vi "PicoErrorHandler2.vi"(8 "error in (no error)":errorcluster={"status"=TRUE, "code"=1, "source"="Default Error In"}, 10 "Default handle":i16=16384, 11 "handle In":i16=16384) -> (0 "error out":errorcluster={"status"=TRUE, "code"=1, "source"="Default Error Out"})   [LabVIEW 2020]
doc: "This VI takes an error cluster and if an error has occurred, displays a message box indicating the source of the error and the status code returned by the driver."
uses:
  ps3000a.dll
  ps2000.dll
  ps4000.dll
  ps5000.dll
  ps3000.dll
  ps6000a.dll
  UsbPT104.dll
  ps2000a.dll
  ps5000a.dll
  ps4000a.dll
  ps6000.dll
  plcm3.dll
panel:
  out "CloseUnit Statuses":T1
  out "Pass or Unknown string":string
  out "Error String":string
  out "handle out":i16=16384
  in  "no error":errorcluster
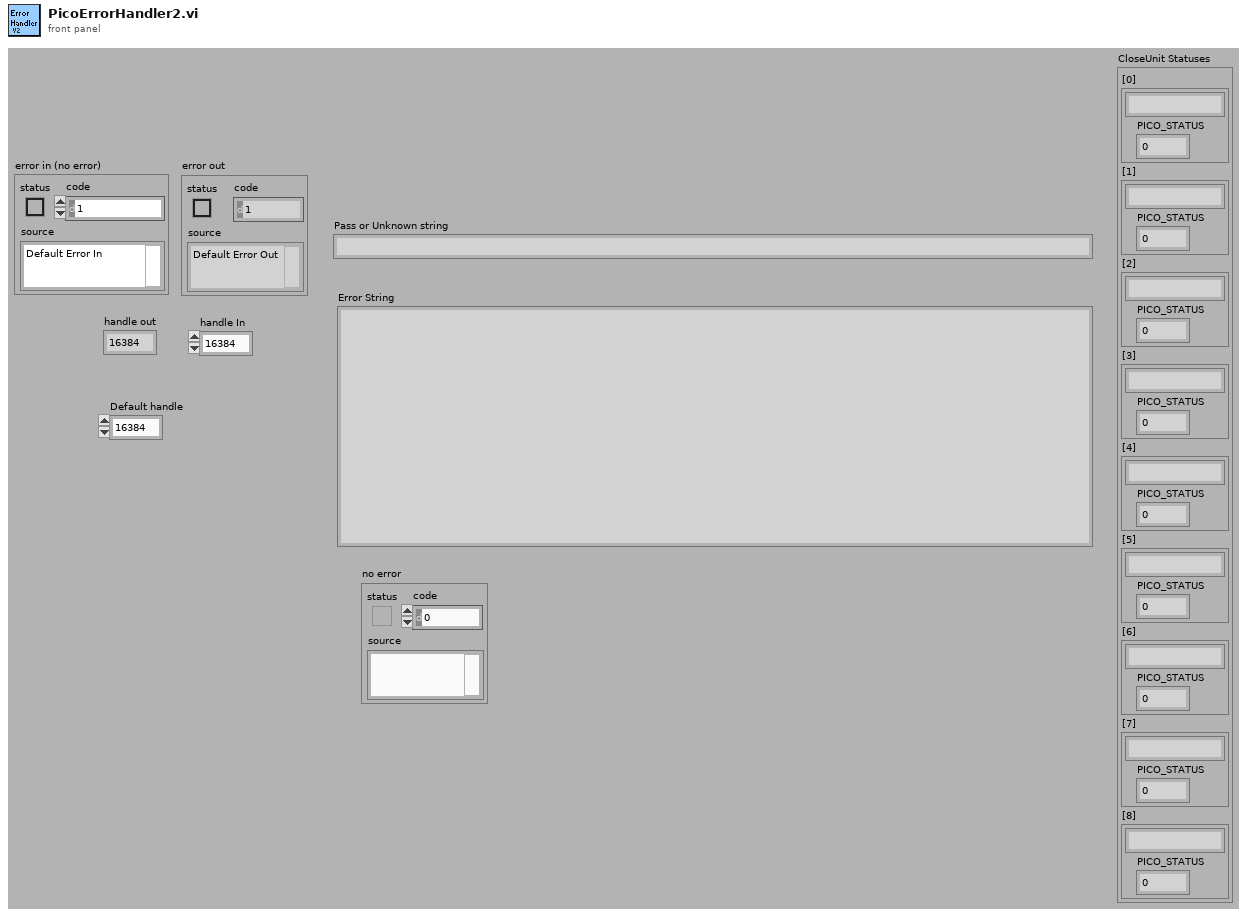
[diagram p1: front panel]
types:
  T1 = cluster{"[0]":cluster{string, "PICO_STATUS":u32}, "[1]":cluster{string, "PICO_STATUS":u32}, "[2]":cluster{string, "PICO_STATUS":u32}, "[3]":cluster{string, "PICO_STATUS":u32}, "[4]":cluster{string, "PICO_STATUS":u32}, "[5]":cluster{string, "PICO_STATUS":u32}, "[6]":cluster{string, "PICO_STATUS":u32}, "[7]":cluster{string, "PICO_STATUS":u32}, "[8]":cluster{string, "PICO_STATUS":u32}}
  T2 = enum16{"Left Button", "Center Button", "Right Button", "Window Close"}
  T3 = cluster{"[0]":cluster{"source":string, "PICO_STATUS":u32}, "[1]":cluster{"source":string, "PICO_STATUS":u32}, "[2]":cluster{"source":string, "PICO_STATUS":u32}, "[3]":cluster{"source":string, "PICO_STATUS":u32}, "[4]":cluster{"source":string, "PICO_STATUS":u32}, "[5]":cluster{"source":string, "PICO_STATUS":u32}, "[6]":cluster{"source":string, "PICO_STATUS":u32}, "[7]":cluster{"source":string, "PICO_STATUS":u32}, "[8]":cluster{"source":string, "PICO_STATUS":u32}}
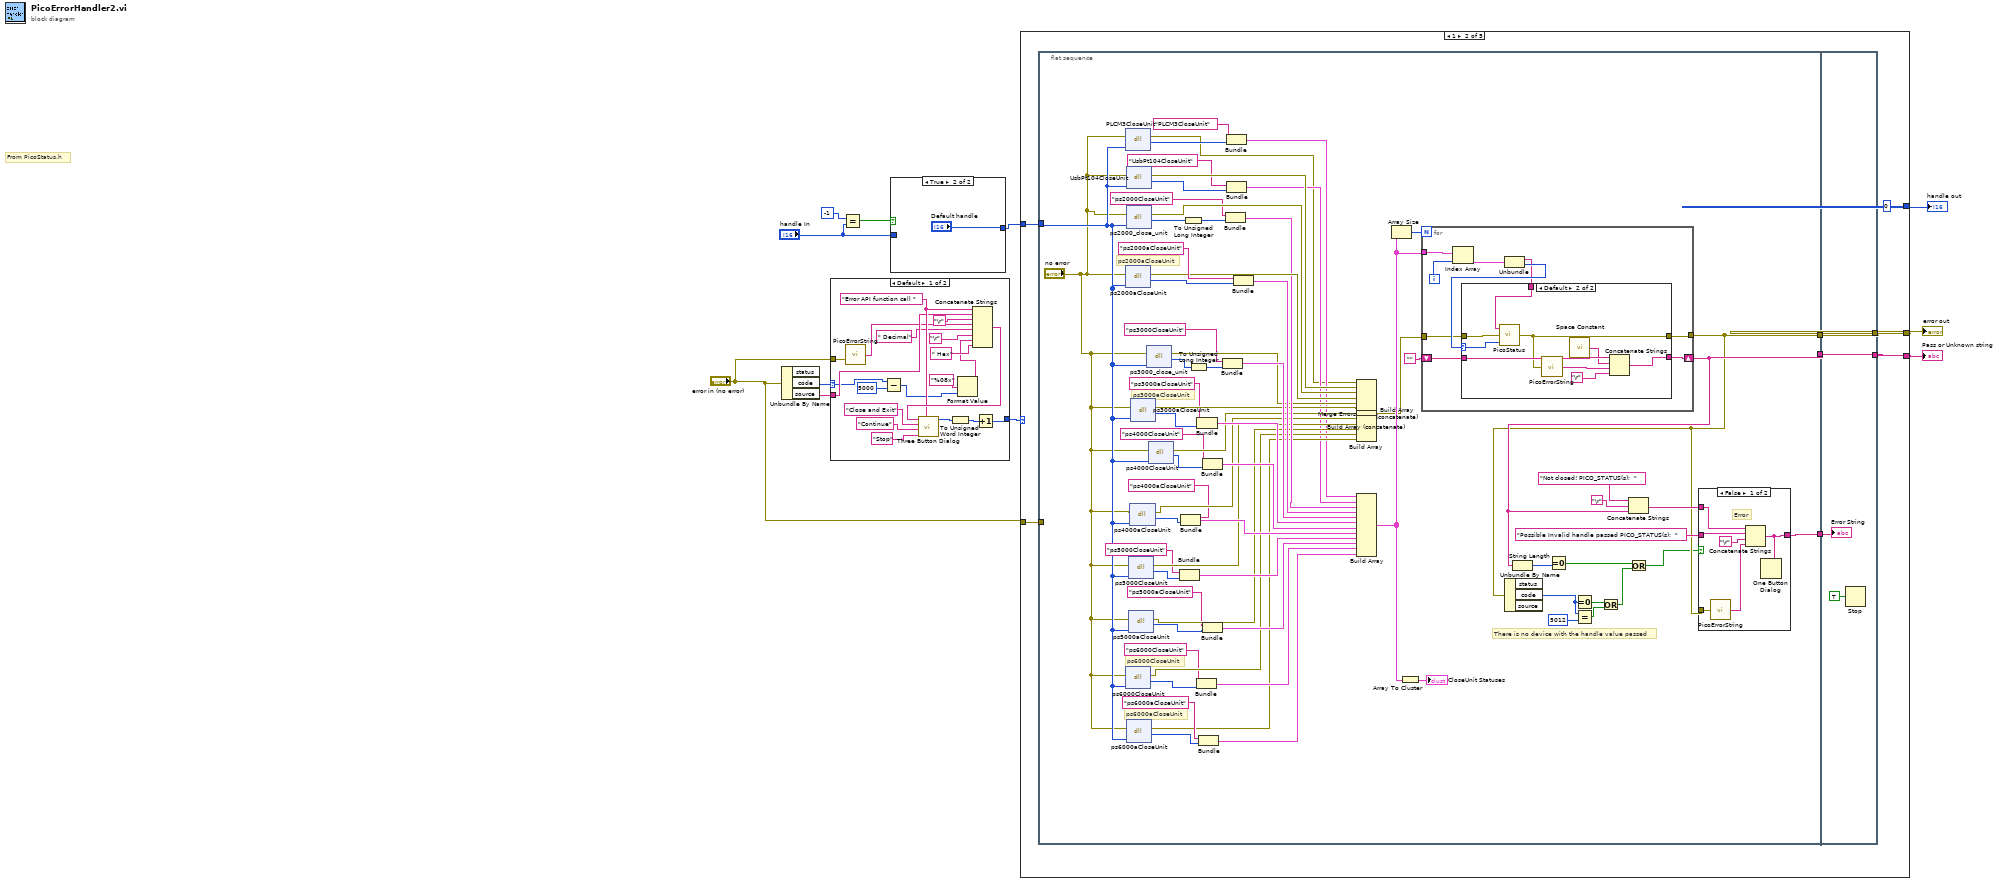
[diagram p0: block diagram]
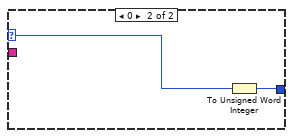
[diagram p3: hidden frame]
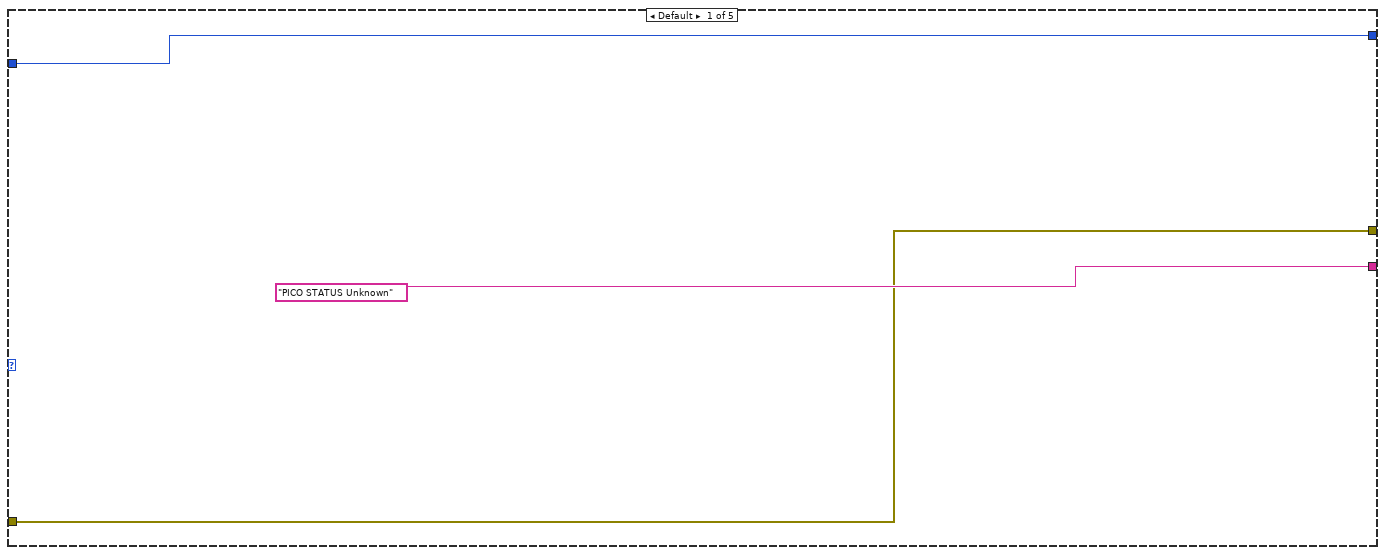
[diagram p4: hidden frame]
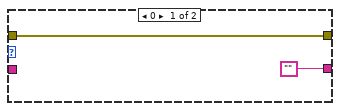
[diagram p6: hidden frame]
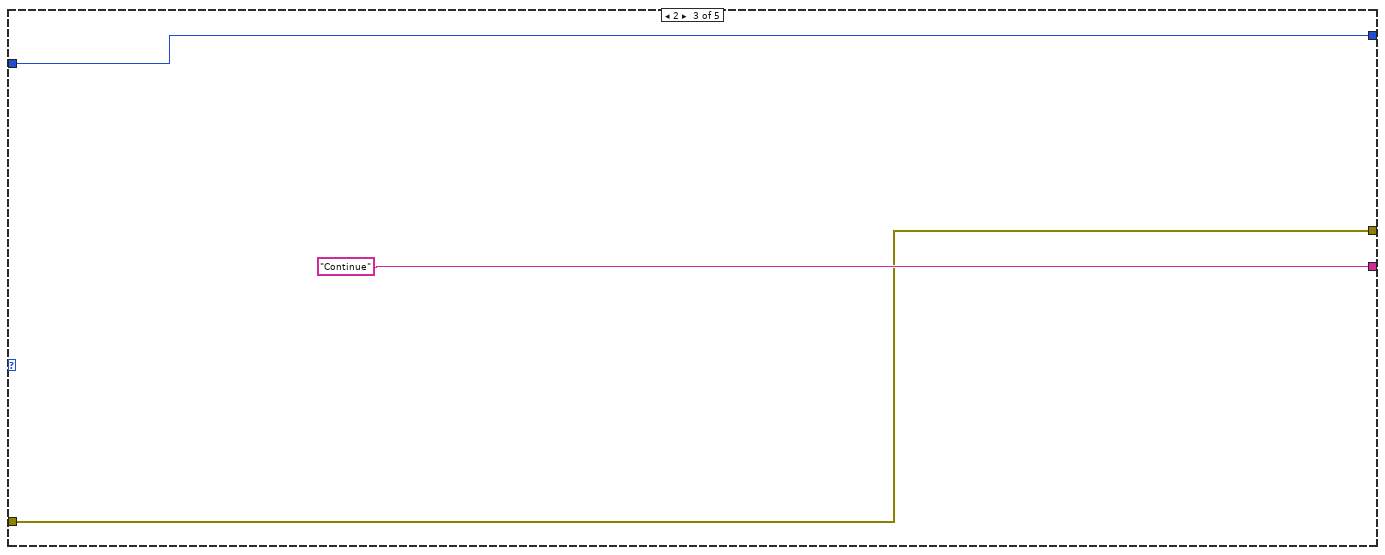
[diagram p7: hidden frame]
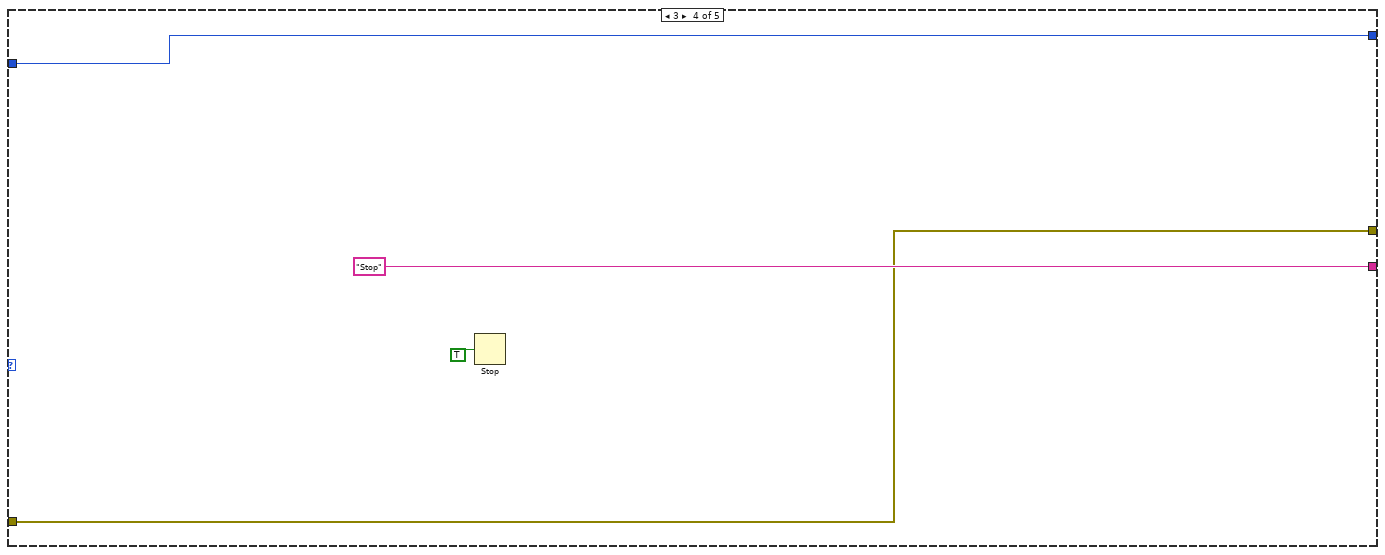
[diagram p8: hidden frame]
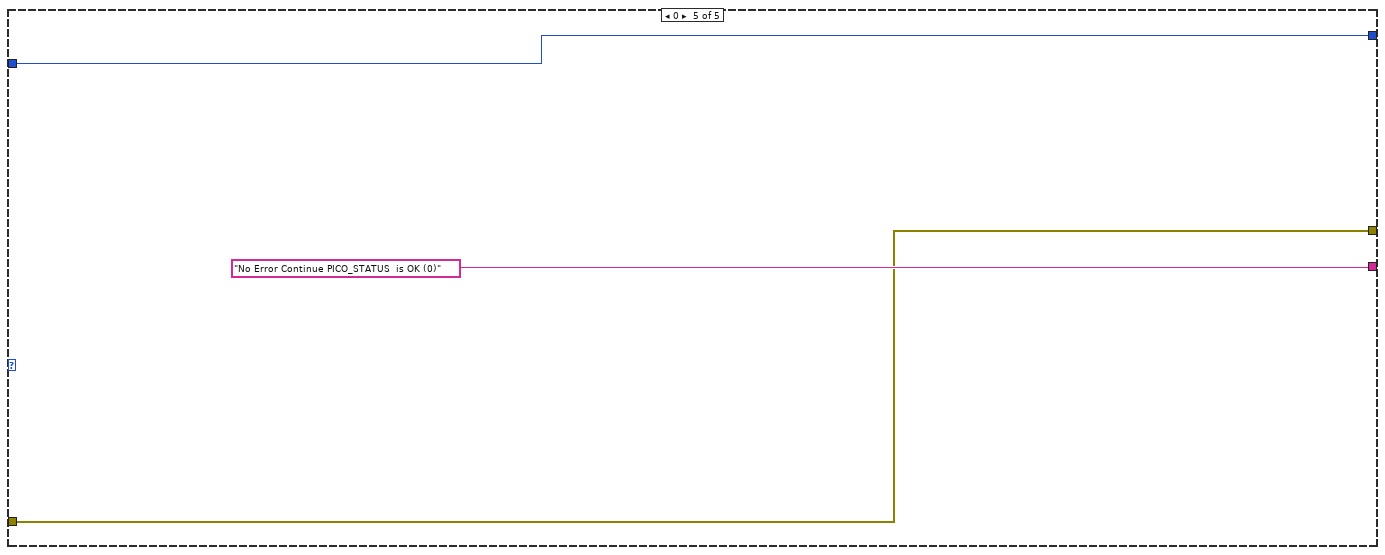
[diagram p9: hidden frame]
diagram:
  # "From PicoStatus.h"
  n1 = Unbundle By Name("error in (no error)") -> ("code"=w10:i32, "source"=w11:string)  [unwired: 1 out]
  n2 = case shown="Default" w10 {
    selector: w10 -> [w16 w32]
    tunnel: w11 -> [w23 _]
    tunnel: [w26 w33] -> w8
    tunnel: "error in (no error)" -> [w21 _]
    frame Default {
      w27 = "Error API function call "
      n3 = call "PicoErrorString.vi"("error in"=w21) -> ("String"=w20:string)  [unwired: 2 in, 2 out]
      n4 = Subtract(x=w16, y=5000) -> (x-y=w19:i32)
      n5 = Format Value(format string="%08x", value (0)=w19) -> (output string=w14:string)  [unwired: 1 in]
      n6 = Concatenate Strings(w27, w23, "\r", w20, " Decimal", "\r", w14, " Hex") -> (w28:string)
      n7 = call <vilib>:"Three Button Dialog.vi"("Window Title (\"\")"=w27, "Right Button Text (\"Cancel\")"="Stop" ("Right Button Text (\"Cancel\")"), "Center Button Text (\"No\")"="Continue" ("Center Button Text (\"No\")"), "Left Button Text (\"Yes\")"="Close and Exit" ("Left Button Text (\"Yes\")"), "message"=w28) -> ("Which Button?"=w24:T2)  [unwired: 6 in]
      n8 = To Unsigned Word Integer(number=w24) -> (unsigned 16bit integer=w25:u16)
      n9 = Increment(x=w25) -> (x+1=w26:u16)
    }
    frame 0 {
      n10 = To Unsigned Word Integer(number=w32) -> (unsigned 16bit integer=w33:u16)
    }
  }
  n11 = Equal?(x=i16 -1, y="handle In") -> (x = y?=w4:bool)
  n12 = case shown="True" w4 {
    tunnel: "handle In" -> [w34 _]
    tunnel: [w34 "Default handle"] -> w2
    frame False {
    }
    frame True {
    }
  }
  n13 = case shown="1" w8 {
    tunnel: w2 -> [w36 w46 w153 w156 w160]
    tunnel: ["PICO STATUS Unknown" w44 "Continue" ("Center Button Text (\"No\")") "Stop" ("Right Button Text (\"Cancel\")") "No Error Continue PICO_STATUS  is OK (0)" ("Center Button Text (\"No\")")] -> w6
    tunnel: [w37 w43 w154 w158 w161] -> w9
    tunnel: "error in (no error)" -> [w37 w45 w154 w158 w161]
    tunnel: [w36 i16 0 ("handle In") w153 w156 w160] -> w7
    frame Default {
    }
    frame 1 {
      n14 = flat-sequence {
        tunnel: w46 -> [w53]
        tunnel: w45 -> [_]
        tunnel: [w114] -> w42
        tunnel: [w71] -> w41
        tunnel: [w112] -> w40
        tunnel: [w151] -> w43
        tunnel: [w152] -> w44
        tunnel: w42 -> [w152]
        tunnel: w41 -> [w151]
        tunnel: w40 -> [w149]
        frame #0 {
          # "ps6000aCloseUnit"
          # "ps6000CloseUnit"
          # "ps3000aCloseUnit"
          # "There is no device with the handle value passed"
          # "ps2000aCloseUnit"
          n15 = dll-call lib="plcm3.dll" fn="PLCM3CloseUnit"(error in="no error", "handle"=w53) -> (error out=w48:errorcluster, "PICO_STATUS"=w51:u32)  [unwired: 3 in, 1 out]
          n16 = dll-call lib="ps2000a.dll" fn="ps2000aCloseUnit" ("ps3000.dll:_ps3000_open_unit@0")(error in="no error", "handle"=w53) -> (error out=w118:errorcluster, "PICO_STATUS"=w58:u32)  [unwired: 3 in, 1 out]
          n17 = dll-call lib="PS6000.dll" fn="ps6000CloseUnit" ("ps3000.dll:_ps3000_open_unit@0")(error in="no error", "handle"=w53) -> (error out=w93:errorcluster, "PICO_STATUS"=w54:u32)  [unwired: 3 in, 1 out]
          n18 = dll-call lib="UsbPT104.dll" fn="UsbPt104CloseUnit"(error in="no error", "handle"=w53) -> (error out=w62:errorcluster, "PICO_STATUS"=w60:u32)  [unwired: 3 in, 1 out]
          n19 = dll-call lib="ps2000.dll" fn="ps2000_close_unit"(error in="no error", "handle"=w53) -> (error out=w91:errorcluster, "return"=w84:i16)  [unwired: 3 in, 1 out]
          n20 = dll-call lib="ps6000a.dll" fn="ps6000aCloseUnit"(error in="no error", "handle"=w53) -> (error out=w63:errorcluster, "PICO_STATUS"=w57:u32)  [unwired: 3 in, 1 out]
          n21 = dll-call lib="ps5000a.dll" fn="ps5000aCloseUnit" ("ps3000.dll:_ps3000_open_unit@0")(error in="no error", "handle"=w53) -> (error out=w94:errorcluster, "PICO_STATUS"=w56:u32)  [unwired: 3 in, 1 out]
          n22 = dll-call lib="PS5000.dll" fn="ps5000CloseUnit" ("ps3000.dll:_ps3000_open_unit@0")(error in="no error", "handle"=w53) -> (error out=w95:errorcluster, "PICO_STATUS"=w74:u32)  [unwired: 3 in, 1 out]
          n23 = dll-call lib="ps4000a.dll" fn="ps4000aCloseUnit" ("ps3000.dll:_ps3000_open_unit@0")(error in="no error", "handle"=w53) -> (error out=w96:errorcluster, "PICO_STATUS"=w55:u32)  [unwired: 3 in, 1 out]
          n24 = dll-call lib="ps3000a.dll" fn="ps3000aCloseUnit" ("ps3000.dll:_ps3000_open_unit@0")(error in="no error", "handle"=w53) -> (error out=w98:errorcluster, "PICO_STATUS"=w83:u32)  [unwired: 3 in, 1 out]
          n25 = dll-call lib="ps3000.dll" fn="ps3000_close_unit" label="CloseUnit"(error in="no error", "handle"=w53) -> (error out=w99:errorcluster, "status"=w72:i16)  [unwired: 3 in, 1 out]
          n26 = dll-call lib="ps4000.dll" fn="ps4000CloseUnit" ("ps3000.dll:_ps3000_open_unit@0")(error in="no error", "handle"=w53) -> (error out=w97:errorcluster, "PICO_STATUS"=w76:u32)  [unwired: 3 in, 1 out]
          n27 = Bundle("ps5000CloseUnit", "PICO_STATUS"=w74) -> (w103:cluster{string, "PICO_STATUS":u32})  [unwired: 1 in]
          n28 = Bundle("ps4000aCloseUnit", "PICO_STATUS"=w55) -> (w104:cluster{string, "PICO_STATUS":u32})  [unwired: 1 in]
          n29 = To Unsigned Long Integer(number=w84) -> (unsigned 32bit integer=w85:u32)
          n30 = To Unsigned Long Integer(number=w72) -> (unsigned 32bit integer=w73:u32)
          n31 = Bundle("ps6000CloseUnit", "PICO_STATUS"=w54) -> (w101:cluster{string, "PICO_STATUS":u32})  [unwired: 1 in]
          n32 = Bundle("ps3000aCloseUnit", "PICO_STATUS"=w83) -> (w106:cluster{string, "PICO_STATUS":u32})  [unwired: 1 in]
          n33 = Bundle("source"="ps6000aCloseUnit", "PICO_STATUS"=w57) -> (w64:cluster{"source":string, "PICO_STATUS":u32})  [unwired: 1 in]
          n34 = Bundle("ps4000CloseUnit", "PICO_STATUS"=w76) -> (w105:cluster{string, "PICO_STATUS":u32})  [unwired: 1 in]
          n35 = Bundle("ps5000aCloseUnit", "PICO_STATUS"=w56) -> (w102:cluster{string, "PICO_STATUS":u32})  [unwired: 1 in]
          n36 = Bundle("ps3000CloseUnit", w73) -> (w107:cluster{string, u32})  [unwired: 1 in]
          n37 = Bundle("ps2000CloseUnit", w85) -> (w109:cluster{string, u32})  [unwired: 1 in]
          n38 = Bundle("PLCM3CloseUnit", "PICO_STATUS"=w51) -> (w49:cluster{string, "PICO_STATUS":u32})  [unwired: 1 in]
          n39 = Bundle("UsbPt104CloseUnit", "PICO_STATUS"=w60) -> (w59:cluster{string, "PICO_STATUS":u32})  [unwired: 1 in]
          n40 = Bundle("ps2000aCloseUnit", "PICO_STATUS"=w58) -> (w108:cluster{string, "PICO_STATUS":u32})  [unwired: 1 in]
          n41 = Build Array(w48, w62, w91, w118, w99, w98, w97, w96, w95, w94, w93, w63) -> (w70:errorcluster[])
          n42 = Build Array (concatenate)(w70) -> (w66:errorcluster[])
          n43 = Build Array (concatenate)(w66) -> (w47:errorcluster[])
          n44 = Merge Errors(w47) -> (w117:errorcluster)
          n45 = Build Array(w49, w59, w109, w108, w107, w106, w105, w104, w103, w102, w101, w64) -> (w120:cluster{"source":string, "PICO_STATUS":u32}[])
          n46 = Array Size(array=w120) -> (size(s)=w92:i32)
          n47 = Array To Cluster(array=w120) -> (cluster=→"CloseUnit Statuses":T3)
          n48 = for {
            N: w92 -> [_]
            shift-right: [w132] -> w114
            shift-left: "" -> [w133]
            tunnel: w120 -> [w137]
            tunnel: w117 -> [w131]
            tunnel: [w130] -> w71
            i -> [w136]
            n49 = Index Array(array=w137, index=w136) -> (element=w135:cluster{"source":string, "PICO_STATUS":u32})
            n50 = Unbundle(w135) -> ("source"=w129:string, "PICO_STATUS"=w134:u32)
            n51 = case shown="Default" w134 {
              selector: w134 -> [_ w147]
              tunnel: ["" w148] -> w132
              tunnel: w133 -> [_ w146]
              tunnel: w131 -> [w138 w142]
              tunnel: [w138 w141] -> w130
              tunnel: w129 -> [_ w140]
              frame 0 {
              }
              frame Default {
                n52 = call "PicoStatus.vi"("PICO STATUS"=w147, "error in"=w142, "source"=w140) -> ("error out"=w141:errorcluster)
                n53 = call "PicoErrorString.vi"("error in"=w141) -> ("String"=w144:string)  [unwired: 2 in, 2 out]
                n54 = call <vilib>:"Space Constant.vi"() -> ("String"=w145:string)
                n55 = Concatenate Strings(w146, w145, w144, "\r") -> (w148:string)
              }
            }
          }
          n56 = Unbundle By Name(w71) -> ("code"=w87:i32)  [unwired: 2 out]
          n57 = String Length(string=w114) -> (length=w113:i32)
          n58 = Equal To 0?(x=w113) -> (x = 0?=w68:bool)
          n59 = Equal To 0?(x=w87) -> (x = 0?=w90:bool)
          n60 = Equal?(x=w87, y=5012) -> (x = y?=w89:bool)
          n61 = Or(x=w90, y=w89) -> (x .or. y?=w69:bool)
          n62 = Concatenate Strings("Not closed! PICO_STATUS(s);  " ("Left Button Text (\"Yes\")"), "\r", w114) -> (w111:string)
          n63 = Or(x=w68, y=w69) -> (x .or. y?=w67:bool)
          n64 = case shown="False" w67 {
            tunnel: [w122 w128] -> w112
            tunnel: w111 -> [w126 w128]
            tunnel: "Possible Invalid handle passed PICO_STATUS(s);  " ("Left Button Text (\"Yes\")") -> [w125 _]
            tunnel: w71 -> [w124 _]
            frame False {
              # "Error"
              n65 = call "PicoErrorString.vi"("error in"=w124) -> ("String"=w123:string)  [unwired: 2 in, 2 out]
              n66 = Concatenate Strings(w126, w125, "\r", w123) -> (w122:string)
              n67 = One Button Dialog(message=w122) -> ()  [unwired: 1 in, 1 out]
            }
            frame True {
            }
          }
        }
        frame #1 {
          n68 = Stop(stop? (T)=TRUE) -> ()
          "Error String" <- w149
        }
      }
    }
    frame 2 {
    }
    frame 3 {
      n69 = Stop(stop? (T)=TRUE) -> ()
    }
    frame 0 {
    }
  }
  "error out" <- w9
  "handle out" <- w7
  "Pass or Unknown string" <- w6
